vi "E1_ExamenDiagnostico.vi"() -> ()   [LabVIEW 2025]
panel:
  out "Numeric":i32
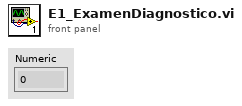
[diagram p1: front panel]
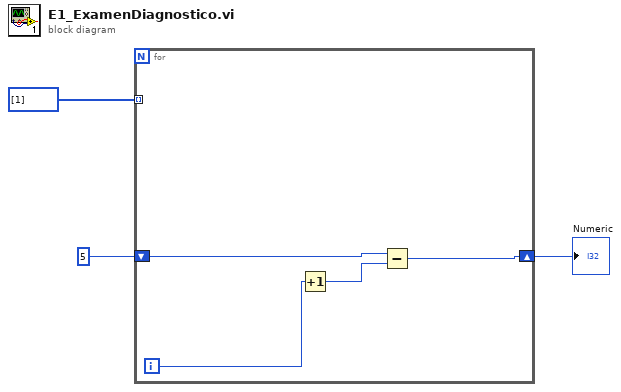
[diagram p0: block diagram]
diagram:
  n1 = for {
    shift-right: [w5] -> w1
    shift-left: 5 -> [w4]
    tunnel: i32[] [1] -> [_] mode=indexing
    i -> [w7]
    n2 = Increment(x=w7) -> (x+1=w6:i32)
    n3 = Subtract(x=w4, y=w6) -> (x-y=w5:i32)
  }
  "Numeric" <- w1
